vi "Retrieve Airmar Data.vi"(8 "error in":errorcluster, 11 "tCRD in":refnum<class "Open Path CRD.lvclass">) -> (0 "error out":errorcluster, 3 "tCRD out":refnum<class "Open Path CRD.lvclass">)   [LabVIEW 2015, in "Open Path CRD.lvclass"]
uses:
  Open Path CRD.lvclass
  Data/Open Path Data.lvclass
  Reusable/CRDS/Main/CRDS.lvclass
  Reusable/CRDS/Data/Cell/CRDS Cell Data.lvclass
  Reusable/CRDS/Cell/CRDS Cell.lvclass
  Reusable/CRDS/Data/Main/CRDS Data.lvclass
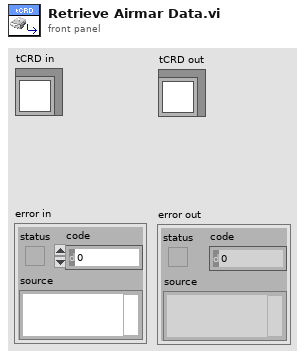
[diagram p1: front panel]
types:
  T1 = typedef "calData.ctl" = cluster{"rhDilFac":sgl, "Q":sgl, "Tmean":sgl, "extDilFac":sgl, "rhCell":sgl, "P":sgl, "T":sgl}
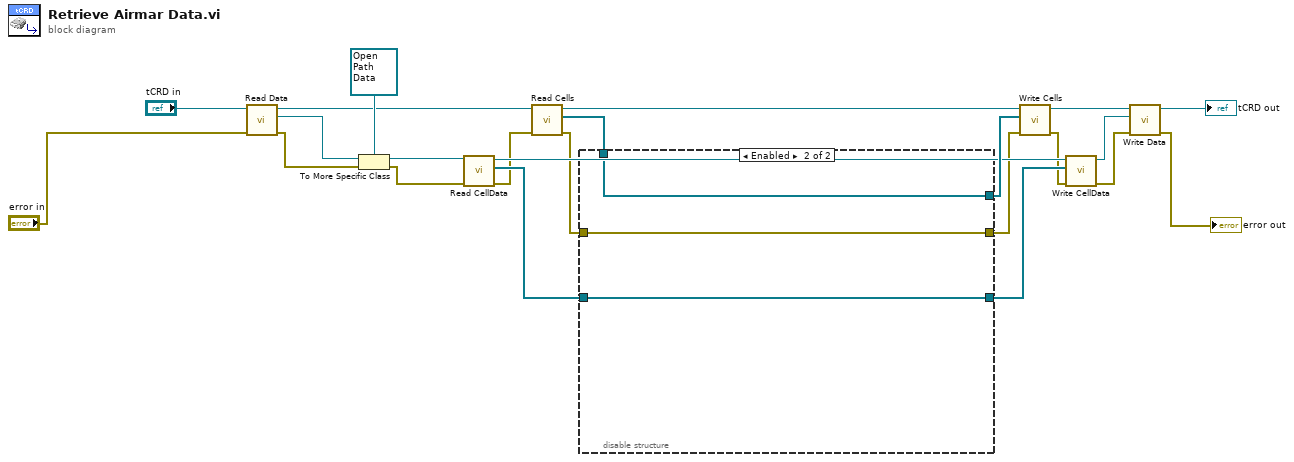
[diagram p0: block diagram]
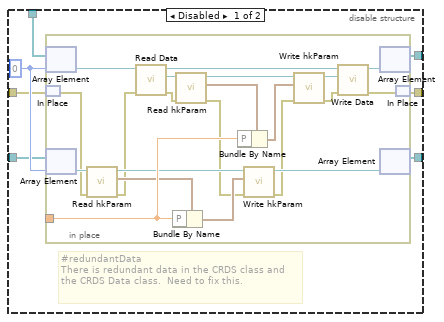
[diagram p2: hidden frame]
diagram:
  n1 = call "Read Data.vi"("error in (no error)"="error in", "CRDS in"="tCRD in") -> ("error out"=w16:errorcluster, "CRDS"=w19:refnum<class "CRDS Data.lvclass">, "CRDS out"=w15:refnum<class "Open Path CRD.lvclass">)  [unwired: 7 in]
  n2 = To More Specific Class(target class=refnum<class "Open Path Data.lvclass"> refnum ("tCRD Data"), reference=w19, error in=w16) -> (specific class reference=w17:refnum<class "Open Path Data.lvclass">, error out=w1:errorcluster)
  n3 = call "Read CellData.vi"("error in"=w1, "CRDS Data in"=w17) -> ("error out"=w6:errorcluster, "CellData"=w7:refnum<class "CRDS Cell Data.lvclass">[], "CRDS Data out"=w8:refnum<class "Open Path Data.lvclass">)  [unwired: 7 in]
  n4 = call "Read Cells.vi"("error in (no error)"=w6, "CRDS in"=w15) -> ("error out"=w4:errorcluster, "Cells"=w12:refnum<class "CRDS Cell.lvclass">[], "CRDS out"=w14:refnum<class "Open Path CRD.lvclass">)  [unwired: 7 in]
  n5 = disable-structure shown="Enabled" {
    disable-tunnel: w12 -> [w30 w54]
    disable-tunnel: [w28 w54] -> w11
    disable-tunnel: [w27 w53] -> w10
    disable-tunnel: w7 -> [w26 w53]
    disable-tunnel: w4 -> [w25 w52]
    disable-tunnel: [w24 w52] -> w3
    frame Disabled {
      w29 = 0
      # "#redundantData\nThere is redundant data in the CRDS class and the CRDS Data class.  Need to fix this."
      n6 = in-place {
        in-place-border: _ -> [w45]
        n7 = in-place-array #1(w30, w29) -> (w51:refnum<class "CRDS Cell.lvclass">)
        n8 = in-place-match #2(w25) -> (w32:errorcluster)
        n9 = in-place-array #3(w26, w29) -> (w40:refnum<class "CRDS Cell Data.lvclass">)
        n10 = call "Read hkParam.vi"("error in"=w32, "CRDS Cell Data in"=w40) -> ("error out"=w35:errorcluster, "hkParam"=w39:T1, "CRDS Cell Data out"=w37:refnum<class "CRDS Cell Data.lvclass">)  [unwired: 7 in]
        n11 = call "Read Data.vi"("error in"=w35, "CRDS Cell in"=w51) -> ("error out"=w41:errorcluster, "CRDS Cell"=w50:refnum<class "CRDS Cell Data.lvclass">, "CRDS Cell out"=w48:refnum<class "CRDS Cell.lvclass">)  [unwired: 7 in]
        n12 = Bundle By Name(cluster=w39, "P"=w45) -> (w38:T1)
        n13 = call "Read hkParam.vi"("error in"=w41, "CRDS Cell Data in"=w50) -> ("error out"=w34:errorcluster, "hkParam"=w44:T1, "CRDS Cell Data out"=w49:refnum<class "CRDS Cell Data.lvclass">)  [unwired: 7 in]
        n14 = Bundle By Name(cluster=w44, "P"=w45) -> (w43:T1)
        n15 = call "Write hkParam.vi"("error in (no error)"=w34, "hkParam"=w38, "CRDS Cell Data in"=w37) -> ("error out"=w33:errorcluster, "CRDS Cell Data out"=w36:refnum<class "CRDS Cell Data.lvclass">)  [unwired: 7 in]
        n16 = call "Write hkParam.vi"("error in (no error)"=w33, "hkParam"=w43, "CRDS Cell Data in"=w49) -> ("error out"=w42:errorcluster, "CRDS Cell Data out"=w47:refnum<class "CRDS Cell Data.lvclass">)  [unwired: 7 in]
        n17 = call "Write Data.vi"("error in"=w42, "CRDS Cell"=w47, "CRDS Cell in"=w48) -> ("error out"=w31:errorcluster, "CRDS Cell out"=w46:refnum<class "CRDS Cell.lvclass">)  [unwired: 7 in]
        n18 = in-place-array #1(w46) -> (w28:refnum<class "CRDS Cell.lvclass">[])  [unwired: 1 out]
        n19 = in-place-array #3(w36) -> (w27:refnum<class "CRDS Cell Data.lvclass">[])  [unwired: 1 out]
        n20 = in-place-match #2(w31) -> (w24:errorcluster)
      }
    }
    frame Enabled {
    }
  }
  n21 = call "Write Cells.vi"("error in (no error)"=w3, "Cells"=w11, "CRDS in"=w14) -> ("error out"=w2:errorcluster, "CRDS out"=w13:refnum<class "Open Path CRD.lvclass">)  [unwired: 7 in]
  n22 = call "Write CellData.vi"("error in"=w2, "CellData"=w10, "CRDS Data in"=w8) -> ("error out"=w5:errorcluster, "CRDS Data out"=w9:refnum<class "Open Path Data.lvclass">)  [unwired: 7 in]
  n23 = call "Write Data.vi"("error in (no error)"=w5, "CRDS"=w9, "CRDS in"=w13) -> ("error out"=→"error out":errorcluster, "CRDS out"=→"tCRD out":refnum<class "Open Path CRD.lvclass">)  [unwired: 7 in]
